vi "Wheel Axis and Button.vi"(9 "Wheel Button Input":T2, 10 "Raw Wheel Axes":T3, 11 "Action":T1(ring)) -> (1 "Wheel Buttons":T2, 2 "Raw Wheel Axes":T3)   [LabVIEW 2013]
uses:
  TypeDefs/Wheel Axes.ctl
  TypeDefs/Wheel Buttons.ctl
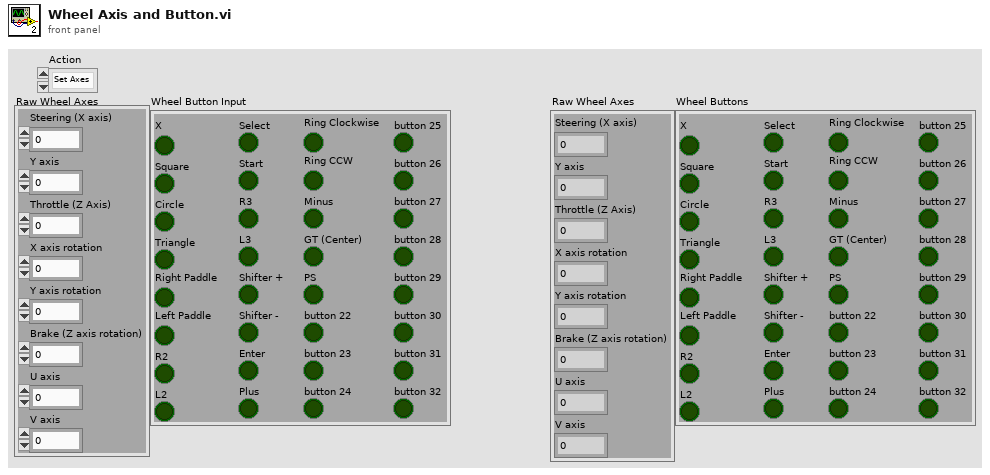
[diagram p1: front panel]
types:
  T1 = enum16{"Set Axes", "Read Axes", "Set Buttons", "Read Buttons", "Get Scaled Throttle", "Get Scaled Steering", "Get Scaled Brake"}
  T2 = typedef "Wheel Buttons.ctl" = cluster{"X":bool, "Square":bool, "Circle":bool, "Triangle":bool, "Right Paddle":bool, "Left Paddle":bool, "R2":bool, "L2":bool, "Select":bool, "Start":bool, "R3":bool, "L3":bool, "Shifter +":bool, "Shifter -":bool, "Enter":bool, "Plus":bool, "Ring Clockwise":bool, "Ring CCW":bool, "Minus":bool, "GT (Center)":bool, "PS":bool, "button 22":bool, "button 23":bool, "button 24":bool, "button 25":bool, "button 26":bool, "button 27":bool, "button 28":bool, "button 29":bool, "button 30":bool, "button 31":bool, "button 32":bool}
  T3 = typedef "Wheel Axes.ctl" = cluster{"Steering (X axis)":i32, "Y axis":i32, "Throttle (Z Axis)":i32, "X axis rotation":i32, "Y axis rotation":i32, "Brake (Z axis rotation)":i32, "U axis":i32, "V axis":i32}
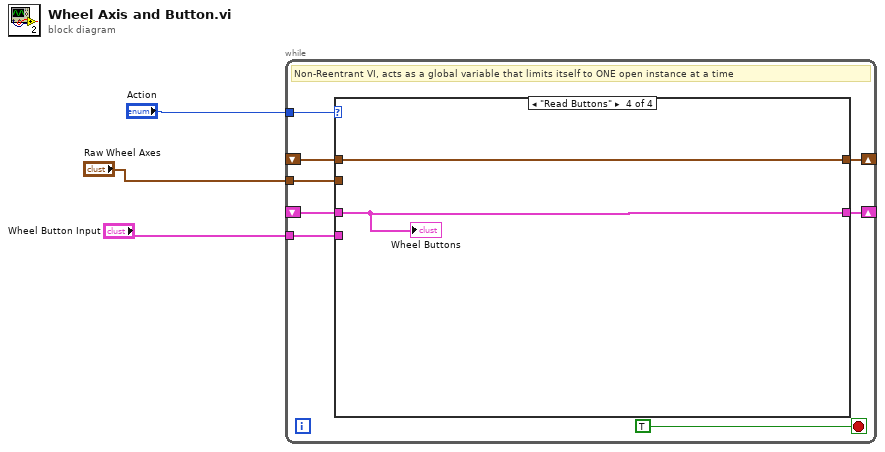
[diagram p0: block diagram]
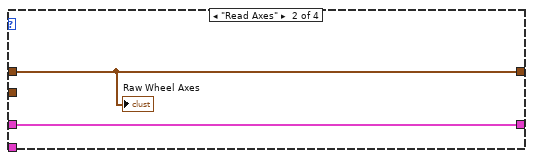
[diagram p3: hidden frame]
diagram:
  n1 = while {
    tunnel: "Action" -> [w10]
    shift-right: [w7] -> _
    shift-left: _ -> [w6]
    shift-right: [w5] -> _
    shift-left: _ -> [w4]
    tunnel: "Raw Wheel Axes" -> [w9]
    tunnel: "Wheel Button Input" -> [w8]
    stop <- TRUE stop-if-true
    # "Non-Reentrant VI, acts as a global variable that limits itself to ONE open instance at a time"
    n2 = case shown="\"Read Buttons\"" w10 {
      tunnel: w9 -> [w13 _ _ _]
      tunnel: w8 -> [_ _ w17 _]
      tunnel: [w13 w15 w16 w19] -> w7
      tunnel: w6 -> [_ w15 w16 w19]
      tunnel: [w12 w14 w17 w18] -> w5
      tunnel: w4 -> [w12 w14 _ w18]
      frame "Set Axes", Default {
      }
      frame "Read Axes" {
        "Raw Wheel Axes" <- w15
      }
      frame "Set Buttons" {
      }
      frame "Read Buttons" {
        "Wheel Buttons" <- w18
      }
    }
  }
